vi "Week2_Slide44_PlotEllipse.vi"() -> ()   [LabVIEW 2015]
panel:
  out "XY Graph":cluster{dbl[], dbl[]}[](graph)
  in  "Minor Axis B":dbl
  in  "Major Axis A":dbl
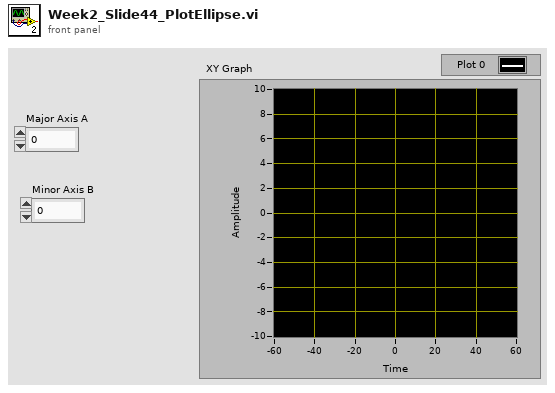
[diagram p1: front panel]
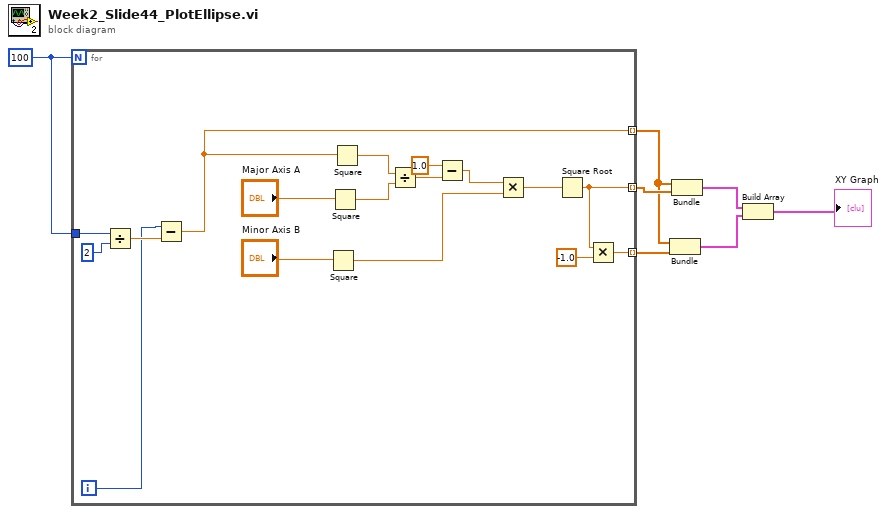
[diagram p0: block diagram]
diagram:
  w6 = 100
  n1 = for {
    N: w6 -> [_]
    tunnel: [w10] -> w7 mode=indexing
    tunnel: w6 -> [w15]
    tunnel: [w11] -> w5 mode=indexing
    tunnel: [w8] -> w4 mode=indexing
    i -> [w12]
    n2 = Divide(x=w15, y=2) -> (x/y=w13:dbl)
    n3 = Subtract(x=w12, y=w13) -> (x-y=w11:dbl)
    n4 = Square(x="Minor Axis B") -> (x^2=w20:dbl)
    n5 = Square(x="Major Axis A") -> (x^2=w23:dbl)
    n6 = Square(x=w11) -> (x^2=w22:dbl)
    n7 = Divide(x=w22, y=w23) -> (x/y=w18:dbl)
    n8 = Subtract(x=1.0, y=w18) -> (x-y=w17:dbl)
    n9 = Multiply(x=w17, y=w20) -> (x*y=w19:dbl)
    n10 = Square Root(x=w19) -> (sqrt(x)=w10:dbl)
    n11 = Multiply(x=w10, y=-1.0) -> (x*y=w8:dbl)
  }
  n12 = Bundle "Bundle"(w5, w4) -> (w2:cluster{dbl[], dbl[]})  [unwired: 1 in]
  n13 = Bundle "Bundle"(w5, w7) -> (w3:cluster{dbl[], dbl[]})  [unwired: 1 in]
  n14 = Build Array "Build Array"(w3, w2) -> (→"XY Graph":cluster{dbl[], dbl[]}[])
